vi "Send TX Message.vi"(8 "error in (no error)":errorcluster, 11 "RxTx in":refnum<class "CCS_RxTx.lvclass">) -> (0 "error out":errorcluster, 3 "RxTx out":refnum<class "CCS_RxTx.lvclass">)   [LabVIEW 2018, in "CCS_RxTx.lvclass"]
doc: "Send Tx message"
uses:
  CCS_RxTx.lvclass
  CCS_RxTx.lvclass/CCS_RxTx.ctl
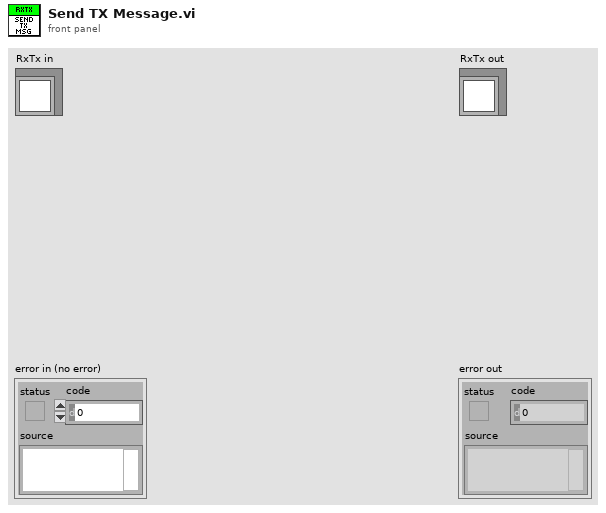
[diagram p1: front panel]
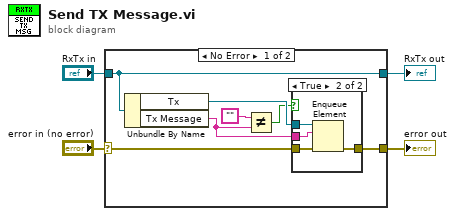
[diagram p0: block diagram]
diagram:
  n1 = case shown="No Error" "error in (no error)" {
    selector: "error in (no error)" -> [w10 w18]
    tunnel: [w8 w18] -> w3
    tunnel: [w9 w17] -> w1
    tunnel: "RxTx in" -> [w9 w17]
    frame No Error {
      n2 = Unbundle By Name(w9) -> ("Tx"=w11:refnum<queue>, "Tx Message"=w7:string)
      n3 = Not Equal?(x="", y=w7) -> (x != y?=w5:bool)
      n4 = case shown="True" w5 {
        tunnel: w11 -> [_ w16]
        tunnel: w10 -> [w12 w15]
        tunnel: [w12 w14] -> w8
        tunnel: w7 -> [_ w13]
        frame False {
        }
        frame True {
          n5 = Enqueue Element(queue=w16, element=w13, error in (no error)=w15) -> (error out=w14:errorcluster)  [unwired: 1 in, 2 out]
        }
      }
    }
    frame Error {
    }
  }
  "error out" <- w3
  "RxTx out" <- w1
